vi "SaveTest.vi"() -> ()   [LabVIEW 2024]
uses:
  836989bf-d2dd-4d25-ac74-3b25aca66eef.vi
  <extravilib>/ChannelInstances/Stream-c(a[.,.](str),a[.,.](str),bool)/Read With Abort.vi
  <extravilib>/ChannelInstances/Stream-c(a[.,.](str),a[.,.](str),bool)/Write With Abort.vi
  <extravilib>/ChannelInstances/Stream-c(a[.,.](str),a[.,.](str),bool)/EndpointRead.vi
  <extravilib>/ChannelInstances/Stream-c(a[.,.](str),a[.,.](str),bool)/Endpoint.vi
  <extravilib>/ChannelInstances/Stream-c(a[.,.](str),a[.,.](str),bool)/Instantiate.vi
  <extravilib>/ChannelInstances/Stream-c(a[.,.](str),a[.,.](str),bool)/)Channel.vi
  <resource>/ChannelSupport/_ChannelSupport/WaitIfNeeded.vi
  <vilib>/Utility/file.llb/Write Delimited Spreadsheet (string).vi
  <extravilib>/ChannelInstances/Stream-c(a[.,.](str),a[.,.](str),bool).lvlib
panel:
  out "Value":string[][](array[string])
  out "Freezing points":string[][](array[string])
  in  "stop":bool
  out "number (0 to 1)":dbl
  out "Freezing data":bool
  in  "Freezing value":sgl
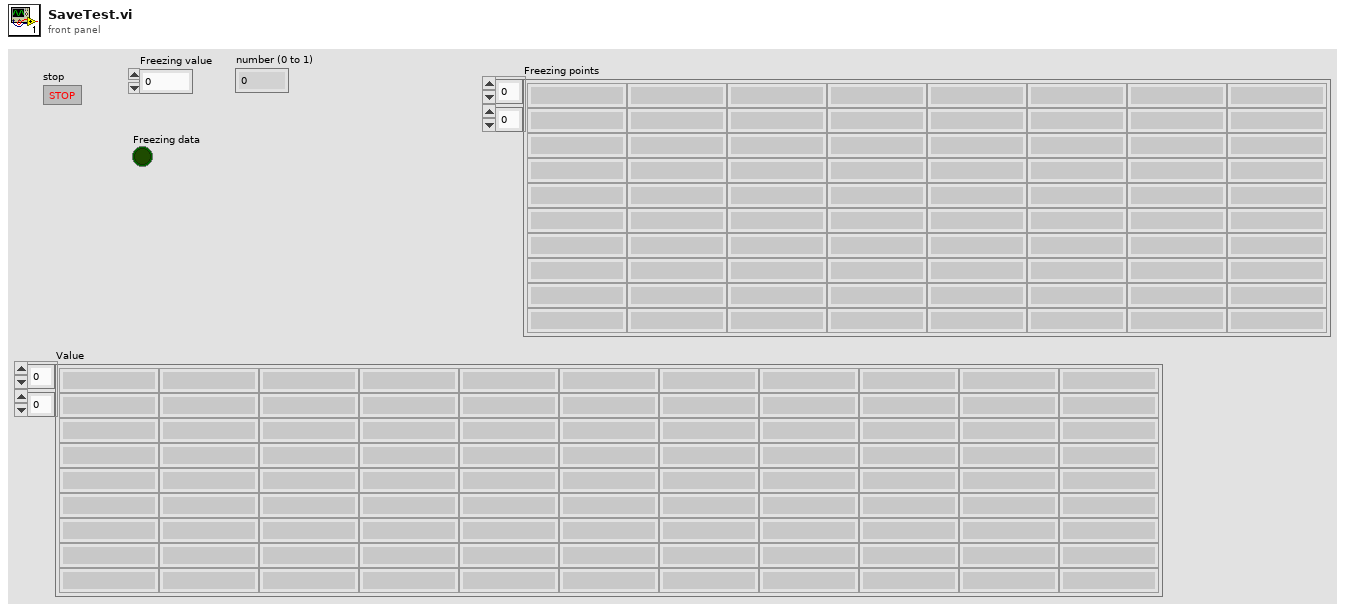
[diagram p1: front panel]
types:
  T1 = cluster{"Freezing points":string[][], "Values":string[][], "Freezing":bool}
  T2 = typedef "Stream-c(a[.,.](str),a[.,.](str),bool).lvlib/)Channel.ctl" = refnum<queue>
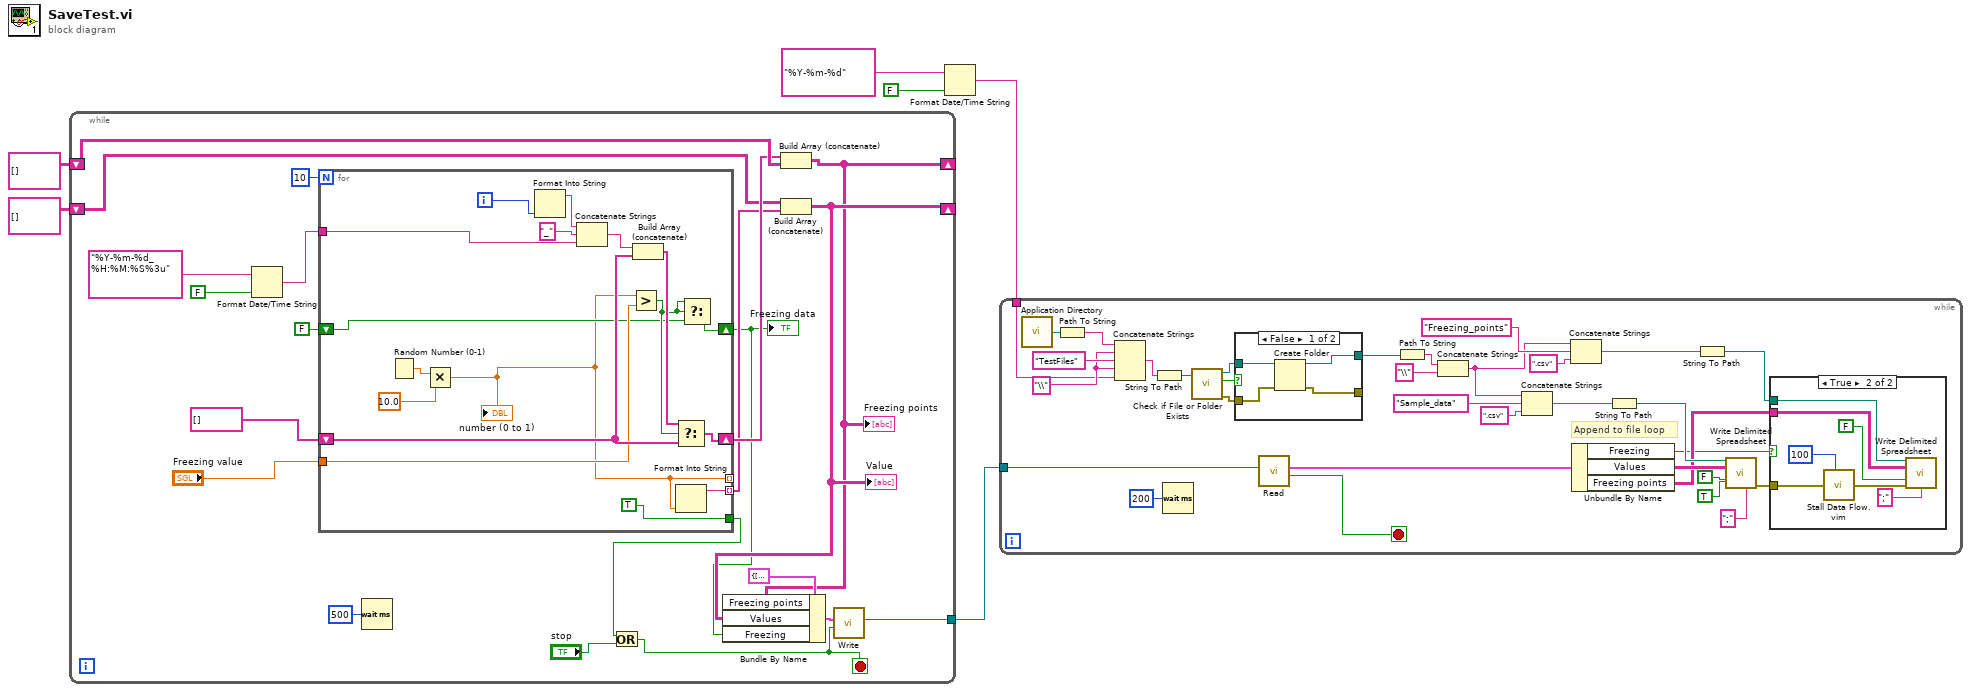
[diagram p0: block diagram]
diagram:
  n1 = while {
    shift-right: [w15] -> _
    shift-left: string[][] [] -> [w25]
    shift-right: [w19] -> _
    shift-left: string[][] [] -> [w23]
    tunnel: [w16] -> w4
    stop <- w9 stop-if-true
    n2 = Format Date/Time String(time format string (%c)="%Y-%m-%d_%H:%M:%S%3u", UTC format=FALSE) -> (date/time string=w12:string)  [unwired: 1 in]
    n3 = for {
      N: 10 -> [_]
      tunnel: [w29] -> _ mode=indexing
      tunnel: [w44] -> w22 mode=indexing
      tunnel: w12 -> [w41]
      shift-right: [w43] -> w24
      shift-left: string[] [] -> [w38]
      tunnel: "Freezing value" -> [w37]
      shift-right: [w33] -> w18
      shift-left: FALSE -> [w32]
      tunnel: [TRUE] -> w7
      i -> [w35]
      n4 = Random Number (0-1)() -> (number: 0 to 1=w31:dbl)
      n5 = Multiply(x=w31, y=10.0) -> (x*y=w29:dbl)
      "number (0 to 1)" <- w29
      n6 = Format Into String(w35) -> (resulting string=w42:string)  [unwired: 3 in, 1 out]
      n7 = Concatenate Strings(w42, "_" ("string"), w41) -> (w40:string)
      n8 = Greater?(x=w29, y=w37) -> (0:w34:bool)
      n9 = Build Array (concatenate)(w40, w38) -> (w39:string[])
      n10 = Select(t=w39, s=w34, f=w38) -> (s? t:f=w43:string[])
      n11 = Format Into String(w29) -> (resulting string=w44:string)  [unwired: 3 in, 1 out]
      n12 = Select(t=w34, s=w34, f=w32) -> (s? t:f=w33:bool)
    }
    "Freezing data" <- w18
    n13 = Wait (ms)(milliseconds to wait=u32 500) -> ()  [unwired: 1 out]
    n14 = Or(x=w7, y="stop") -> (x .or. y?=w9:bool)
    n15 = Build Array (concatenate)(w24, w25) -> (w15:string[][])
    "Freezing points" <- w15
    n16 = Build Array (concatenate)(w23, w22) -> (w19:string[][])
    "Value" <- w19
    n17 = Bundle By Name(cluster=T1 {"Freezing points"=[], "Values"=[], "Freezing"=FALSE}, "Freezing points"=w15, "Values"=w19, "Freezing"=w18) -> (w17:T1)
    n18 = call <extravilib>:"Write.vi"("last element? (F)"=w9, "element"=w17) -> ("channel"=w16:T2)  [unwired: 7 in, 2 out]
  }
  n19 = Format Date/Time String(time format string (%c)="%Y-%m-%d", UTC format=FALSE) -> (date/time string=w1:string)  [unwired: 1 in]
  n20 = while {
    tunnel: w4 -> [w77]
    tunnel: w1 -> [w47]
    stop <- w76 stop-if-true
    w54 = "\\" ("string")
    # "Append to file loop"
    n21 = call <vilib>:"Application Directory.vi"() -> ("Application Directory"=w56:path)
    n22 = Path To String(path=w56) -> (string=w55:string)
    n23 = Concatenate Strings(w55, w54, "TestFiles" ("string"), w54, w47) -> (w51:string)
    n24 = String To Path(string=w51) -> (path=w52:path)
    n25 = Wait (ms)(milliseconds to wait=u32 200) -> ()  [unwired: 1 out]
    n26 = call <vilib>:"Check if File or Folder Exists.vi"("path"=w52) -> ("error out"=w49:errorcluster, "file or folder exists?"=w50:bool, "dup path"=w53:path)  [unwired: 8 in]
    n27 = case shown="False" w50 {
      tunnel: [w81 w83] -> w48
      tunnel: w53 -> [w80 w83]
      tunnel: w49 -> [w79 w82]
      tunnel: [w78 w82] -> _
      frame False {
        n28 = Create Folder(path (use dialog)=w80, error in=w79) -> (created path=w81:path, error out=w78:errorcluster)  [unwired: 1 in, 1 out]
      }
      frame True {
      }
    }
    n29 = call <extravilib>:"Read.vi"("channel"=w77) -> ("last element?"=w76:bool, "element"=w75:T1)  [unwired: 6 in, 3 out]
    n30 = Path To String(path=w48) -> (string=w68:string)
    n31 = Concatenate Strings(w68, "\\" ("string")) -> (w67:string)
    n32 = Concatenate Strings(w67, "Sample_data" ("string"), ".csv" ("string")) -> (w74:string)
    n33 = Concatenate Strings(w67, "Freezing_points" ("string"), ".csv" ("string")) -> (w71:string)
    n34 = Unbundle By Name(w75) -> ("Freezing"=w45:bool, "Values"=w59:string[][], "Freezing points"=w58:string[][])
    n35 = String To Path(string=w74) -> (path=w64:path)
    n36 = String To Path(string=w71) -> (path=w65:path)
    n37 = call-poly <vilib>:"Write Delimited Spreadsheet.vi"("file path (dialog if empty)"=w64, "2D data"=w59, "append to file? (new file:F)"=FALSE, "transpose? (no:F)"=TRUE, "delimiter (\\t)"=";" ("delimiter (\\t)")) -> ("error out"=w62:errorcluster)  [unwired: 9 in, 1 out]
    n38 = case shown="True" w45 {
      tunnel: w65 -> [_ w87]
      tunnel: w62 -> [_ w90]
      tunnel: w58 -> [_ w84]
      frame False {
      }
      frame True {
        n39 = call "Stall Data Flow.vim"("value in"=w90, "milliseconds to wait"=u32 100) -> ("value out"=w88:errorcluster)  [unwired: 1 out]
        n40 = call-poly <vilib>:"Write Delimited Spreadsheet.vi"("file path (dialog if empty)"=w87, "2D data"=w84, "append to file? (new file:F)"=FALSE, "error in (no error)"=w88, "delimiter (\\t)"=";" ("delimiter (\\t)")) -> ()  [unwired: 9 in, 2 out]
      }
    }
  }
